vi "AddTestMethod_CreateDummyObject.vi"(6 "error in":errorcluster, 9 "Wizard":T1) -> (0 "error out":errorcluster, 3 "Cancelled?":bool)   [LabVIEW 2013]
doc: "Use this template to create a wizard dialog."
uses:
  <resource>/Framework/Providers/API/ItemRef.ctl
panel:
  in  "OK Button":bool
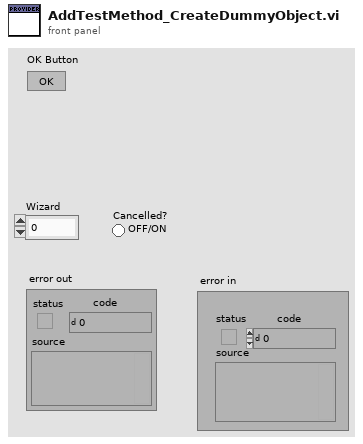
[diagram p1: front panel]
types:
  T1 = typedef "ItemRef.ctl" = u64
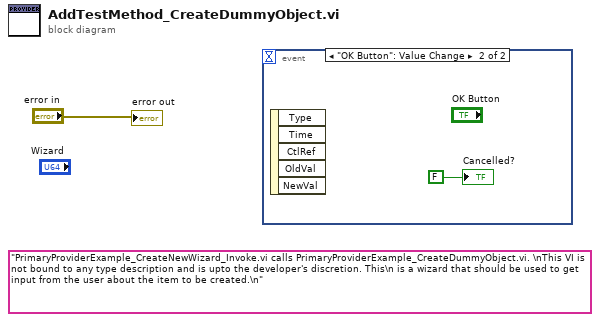
[diagram p0: block diagram]
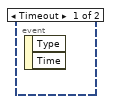
[diagram p2: hidden frame]
diagram:
  (unwired) "PrimaryProviderExample_CreateNewWizard_Invoke.vi calls PrimaryProviderExample_CreateDummyObject.vi. \nThis VI is not bound to any type description and is upto the developer's discretion. This\n is a wizard that should be used to get input from the user about the item to be created.\n" ("message")
  n1 = event shown="[1] \"OK Button\": Value Change" {
    selector: _ -> [_ _]
    dyn-events: _ -> [_ _]
    timeout: _ -> [_ _]
    event Timeout {
      n2 = event-data() -> ()  [unwired: 1 in, 2 out]
    }
    event "OK Button": Value Change {
      n3 = event-data() -> ()  [unwired: 1 in, 5 out]
      "Cancelled?" <- FALSE ("Cancelled?")
    }
  }
  "error out" <- "error in"
